vi "Open PDFStamper.vi"(0 "PDF Path":path, 7 "RotateContents (F)":bool, 11 "error in (no error)":errorcluster) -> (4 "PDFStamper":refnum<k24>, 8 "Temporary File Name":path, 10 "NumberOfPages":i32, 15 "error out":errorcluster)   [LabVIEW 2013]
doc: "Developed by Jean-Marc Simard\nCopyright © 2010, Exaprom Inc.\nAll rights reserved.\nLicense: BSD\n\nWith iTextSharp 4.1.6 (http://itextsharp.sourceforge.net)\nunder Mozilla Public License Version 1.1\n(http://www.mozilla.org/MPL/MPL-1.1.html)"
uses:
  C:/Users/MaxCorp/Documents/GitHub/TopView/DLL/itextsharp.dll
  DLL/itextsharp.dll
  Controls/Temporary Image File.ctl
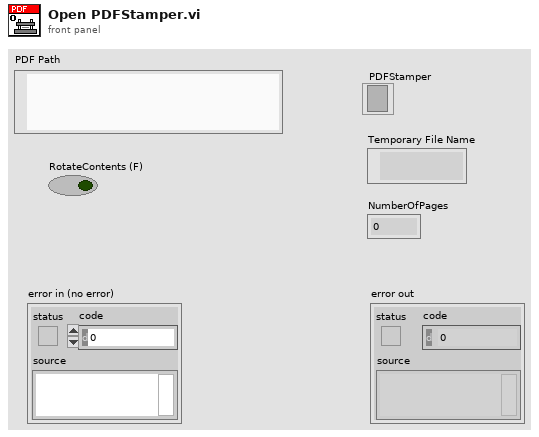
[diagram p1: front panel]
types:
  T1 = typedef "Temporary Image File.ctl" = enum16{".bmp", ".jpeg", ".png", ".pdf", "No File"}
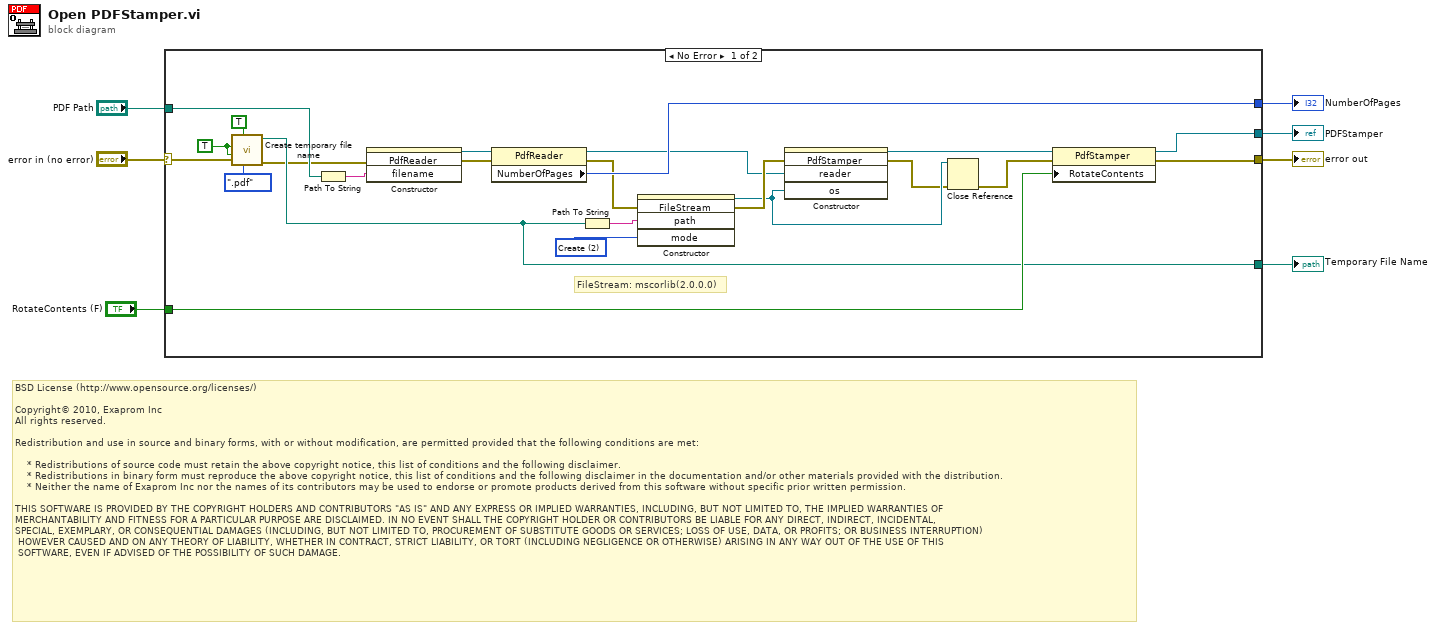
[diagram p0: block diagram]
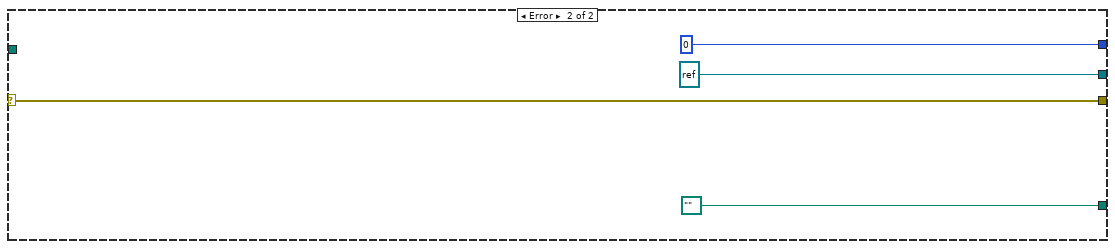
[diagram p2: hidden frame]
diagram:
  # "BSD License (http://www.opensource.org/licenses/)\n\nCopyright© 2010, Exaprom Inc\nAll rights reserved.\n\nRedistribution and use in source and binary forms, with or without modification, are permitted provided that the following conditions are met:\n\n    * Redistributions of source code must retain the above copyright notice, this list of conditions and the following disclaimer.\n    * Redistributions in binary form must reproduce the above copyright notice, this list of conditions and the following disclaimer in the documentation and/or other materials provided with the distribution.\n    * Neither the name of Exaprom Inc nor the names of its contributors may be used to endorse or promote products derived from this software without specific prior written permission.\n\nTHIS SOFTWARE IS PROVIDED BY THE COPYRIGHT HOLDERS AND CONTRIBUTORS \"AS IS\" AND ANY EXPRESS OR IMPLIED WARRANTIES, INCLUDING, BUT NOT LIMITED TO, THE IMPLIED WARRANTIES OF \nMERCHANTABILITY AND FITNESS FOR A PARTICULAR PURPOSE ARE DISCLAIMED. IN NO EVENT SHALL THE COPYRIGHT HOLDER OR CONTRIBUTORS BE LIABLE FOR ANY DIRECT, INDIRECT, INCIDENTAL,\nSPECIAL, EXEMPLARY, OR CONSEQUENTIAL DAMAGES (INCLUDING, BUT NOT LIMITED TO, PROCUREMENT OF SUBSTITUTE GOODS OR SERVICES; LOSS OF USE, DATA, OR PROFITS; OR BUSINESS INTERRUPTION)\n HOWEVER CAUSED AND ON ANY THEORY OF LIABILITY, WHETHER IN CONTRACT, STRICT LIABILITY, OR TORT (INCLUDING NEGLIGENCE OR OTHERWISE) ARISING IN ANY WAY OUT OF THE USE OF THIS\n SOFTWARE, EVEN IF ADVISED OF THE POSSIBILITY OF SUCH DAMAGE."
  n1 = case shown="No Error" "error in (no error)" {
    selector: "error in (no error)" -> [w26 w34]
    tunnel: [w29 w34] -> w5
    tunnel: "PDF Path" -> [w27 _]
    tunnel: [w30 refnum<k24> refnum ("new reference")] -> w3
    tunnel: [w24 0 ("NumberOfPages")] -> w4
    tunnel: "RotateContents (F)" -> [w28 _]
    tunnel: [w25 path "" ("File path")] -> w1
    frame No Error {
      w15 = TRUE ("hh:mm:ss (false)")
      w20 = 2 items=["CreateNew"=1, "Create"=2, "Open"=3, "OpenOrCreate"=4, "Truncate"=5, "Append"=6] ("mode")
      # "FileStream: mscorlib(2.0.0.0)"
      n2 = call "Create temporary file name.vi"("Temporary Image File"=Temporary_Image_File.".pdf", "Flush Files (F)"=TRUE, "error in (no error)"=w26, "msec (F)"=w15, "hh:mm:ss (false)"=w15) -> ("error out"=w13:errorcluster, "File path"=w25:path)  [unwired: 1 in, 4 out]
      n3 = Path To String(path=w27) -> (string=w22:string)
      n4 = constructor class="PdfReader"(error in=w13, "filename"=w22) -> (reference out=w12:refnum<k24>, error out=w19:errorcluster)  [unwired: 2 in, 2 out]
      n5 = property class="PdfReader"(reference=w12, error in=w19) -> (reference out=w10:refnum<k24>, error out=w18:errorcluster, "NumberOfPages"=w24:i32)
      n6 = Path To String(path=w25) -> (string=w21:string)
      n7 = constructor class="FileStream"(error in=w18, "path"=w21, "mode"=w20) -> (reference out=w9:refnum<k24>, error out=w23:errorcluster)  [unwired: 2 in, 3 out]
      n8 = constructor class="PdfStamper"(error in=w23, "reader"=w10, "os"=w9) -> (reference out=w17:refnum<k24>, error out=w8:errorcluster)  [unwired: 2 in, 3 out]
      n9 = Close Reference(reference=w9, error in (no error)=w8) -> (error out=w11:errorcluster)
      n10 = property class="PdfStamper"(reference=w17, error in=w11, "RotateContents"=w28) -> (reference out=w30:refnum<k24>, error out=w29:errorcluster)
    }
    frame Error {
    }
  }
  "error out" <- w5
  "NumberOfPages" <- w4
  "PDFStamper" <- w3
  "Temporary File Name" <- w1
